vi "sns publish to topic.vi"() -> ()   [LabVIEW 2018]
uses:
  Core/HTTP Request/Region.ctl
  Core/HTTP Request/AWS Credentials.ctl
  Topic/Topic.lvclass
  Core/HTTP Request/HTTP Request.lvclass
panel:
  in  "error in (no error)":errorcluster
  out "error out":errorcluster
  in  "AWS Credentials":T1
  in  "Region":T2
  in  "ARN":string
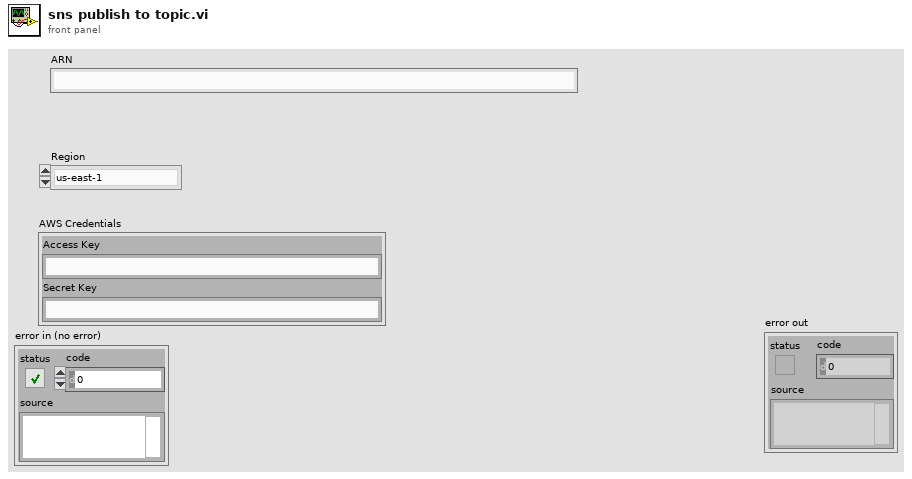
[diagram p1: front panel]
types:
  T1 = typedef "NI_AWS_Core.lvlib/HTTP Request.lvclass/AWS Credentials.ctl" = cluster{"Access Key":string, "Secret Key":string}
  T2 = typedef "NI_AWS_Core.lvlib/HTTP Request.lvclass/Region.ctl" = enum16{"us-east-1", "us-east-2", "us-west-1", "us-west-2", "ap-northeast-1", "ap-northeast-2", "ap-southeast-1", "ap-southeast-2", "ca-central-1", "eu-central-1", "eu-west-1", "eu-west-2", "sa-east-1"}
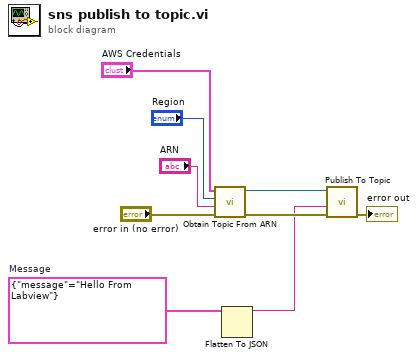
[diagram p0: block diagram]
diagram:
  w4 = cluster{"message":string} {"message"="Hello From Labview"}  # Message
  n1 = call "Obtain Topic From ARN.vi"("error in (no error)"="error in (no error)", "ARN"="ARN", "Region"="Region", "AWS Credentials"="AWS Credentials") -> ("error out"=w6:errorcluster, "Topic"=w5:refnum<class "Topic.lvclass">)  [unwired: 6 in]
  n2 = Flatten To JSON(anything=w4) -> (JSON string=w3:string)  [unwired: 2 in, 1 out]
  n3 = call "Publish To Topic.vi"("error in (no error)"=w6, "Message"=w3, "Topic in"=w5) -> ("error out"=→"error out":errorcluster)  [unwired: 7 in, 1 out]
